vi "Value by Name Key.vi"(11 "Value Name In":string) -> (2 "Value by Name Key":string, 3 "Value Name":string)   [LabVIEW 2020, in "HTTP Server.lvlib" / "Values.lvclass"]
uses:
  Values.lvclass
  Values.lvclass/Values.ctl
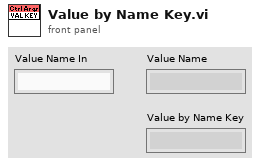
[diagram p1: front panel]
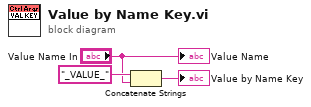
[diagram p0: block diagram]
diagram:
  n1 = Concatenate Strings("_VALUE_" ("string"), "Value Name In") -> (→"Value by Name Key":string)
  "Value Name" <- "Value Name In"
